vi "testCaseRowFormatChk.vi"(8 "error in":errorcluster, 9 "Row number":u32, 10 "Tbl Refnum in":refnum<vi>, 11 "Tree Refnum in":refnum<vi>) -> (0 "error out":errorcluster, 1 "Check result":string="√", 2 "Tbl Refnum out":refnum<vi>, 3 "Tree Refnum out":refnum<vi>)   [LabVIEW 2010]
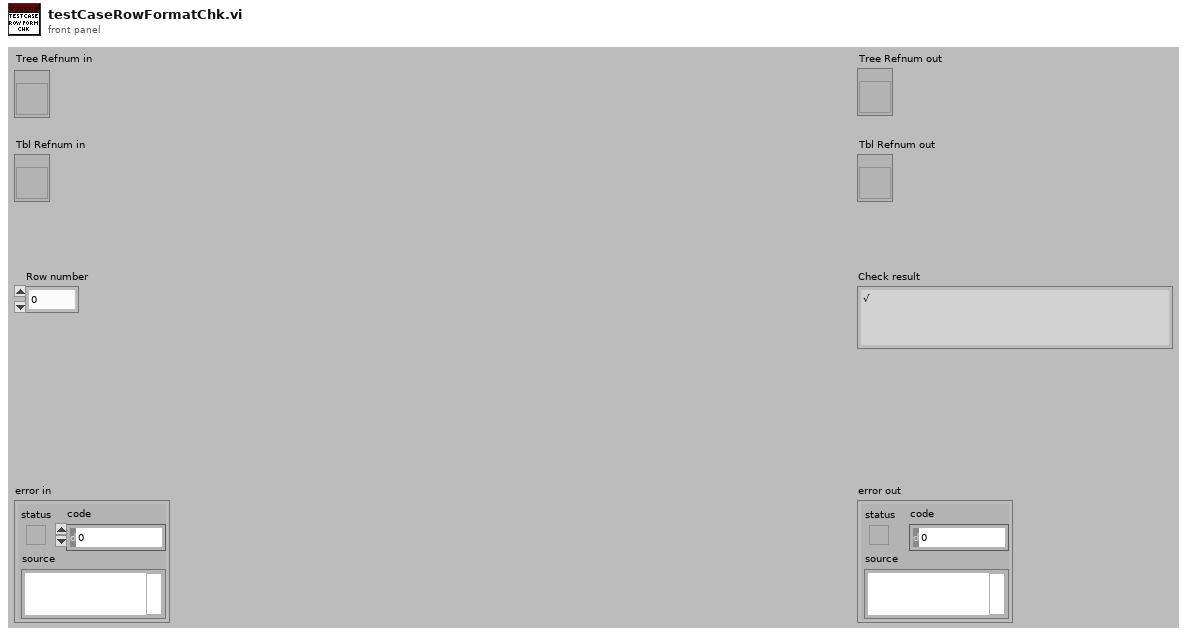
[diagram p1: front panel]
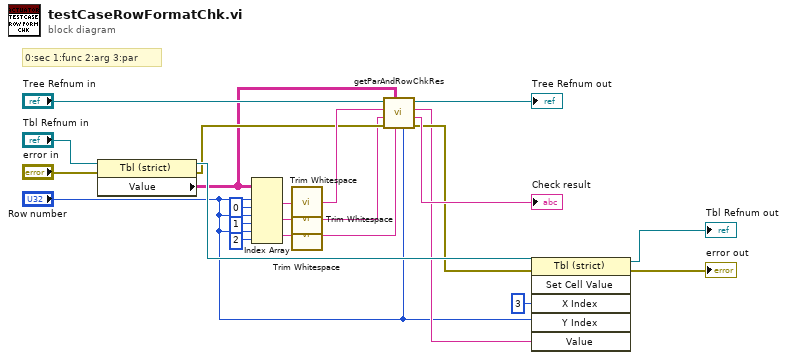
[diagram p0: block diagram]
diagram:
  # "0:sec 1:func 2:arg 3:par"
  n1 = property class="Tbl (strict)"(reference="Tbl Refnum in", error in="error in") -> (reference out=w12:refnum<vi>, error out=w8:errorcluster, "Value"=w1:string[][])
  n2 = Index Array(array=w1, index (row) #1="Row number", index (col) #1=0 ("disabled index (col)"), index (row) #2="Row number", index (col) #2=1 ("index (col)"), index (row) #3="Row number", index (col) #3=2 ("disabled index (col)")) -> (element #1=w21:string, element #2=w19:string, element #3=w17:string)
  n3 = call <vilib>:"Trim Whitespace.vi"("string"=w21) -> ("trimmed string"=w10:string)  [unwired: 1 in]
  n4 = call <vilib>:"Trim Whitespace.vi"("string"=w19) -> ("trimmed string"=w2:string)  [unwired: 1 in]
  n5 = call <vilib>:"Trim Whitespace.vi"("string"=w17) -> ("trimmed string"=w9:string)  [unwired: 1 in]
  n6 = call "getParAndRowChkRes.vi"("Row number"="Row number", "arg"=w9, "table"=w1, "error in"=w8, "function"=w2, "section"=w10, "Tree Refnum in"="Tree Refnum in") -> ("error out"=w5:errorcluster, "Check result"=→"Check result":string, "par"=w4:string, "Tree Refnum out"=→"Tree Refnum out":refnum<vi>)  [unwired: 1 in]
  n7 = invoke class="Tbl (strict)" method="Set Cell Value"(reference=w12, error in=w5, "X Index"=u32 3, "Y Index"="Row number", "Value"=w4) -> (reference out=→"Tbl Refnum out":refnum<vi>, error out=→"error out":errorcluster)  [unwired: 1 in, 4 out]
